vi "FW_PyRunAnnotaion.vi"(0 "Refnum in":refnum<k35>, 5 "python_image":u8[][][](array[numeric]), 9 "appended path":path, 11 "error in (no error)":errorcluster, 12 "Parameters in":T1={"scale_w"=0.0, "scale_h"=0.0, "offset_X"=0.0, "offset_Y"=0.0, "Rho"=0.0, "Theta"=0.0, "Threshold"=14, "min_line_len"=14, "max_line_gap"=30}) -> (1 "2D_image":u8[][](array[numeric]), 3 "elapsed time":u32, 4 "Refnum out":refnum<k35>, 6 "Python_img":u8[][][](array[numeric]), 8 "Lanes":cluster{"X":dbl, "Y":dbl}[][](array[cluster]), 10 "lines":cluster{"X":dbl, "Y":dbl}[][](array[cluster]), 14 "trapezoid_ROI":cluster{"X":dbl, "Y":dbl}[](array[cluster]), 15 "error out":errorcluster)   [LabVIEW 2021, in "Framework_lib.lvlib"]
uses:
  QMH/Framework_lib.lvlib
  FW_pyAnnotation_parameters.ctl
panel:
  out "return value":cluster{"out":dbl, "out 2":i32}
  out "Numeric":u32
  out "input size":cluster{"b":u32, "b":u32, "b":u32}
  # "[[[244 489 383 385]]\n\n [[223 489 380 384]]\n\n [[242 487 304 445]]\n\n [[292 454 370 396]]]"
  # "[[165, 539, 563, 259], []]"
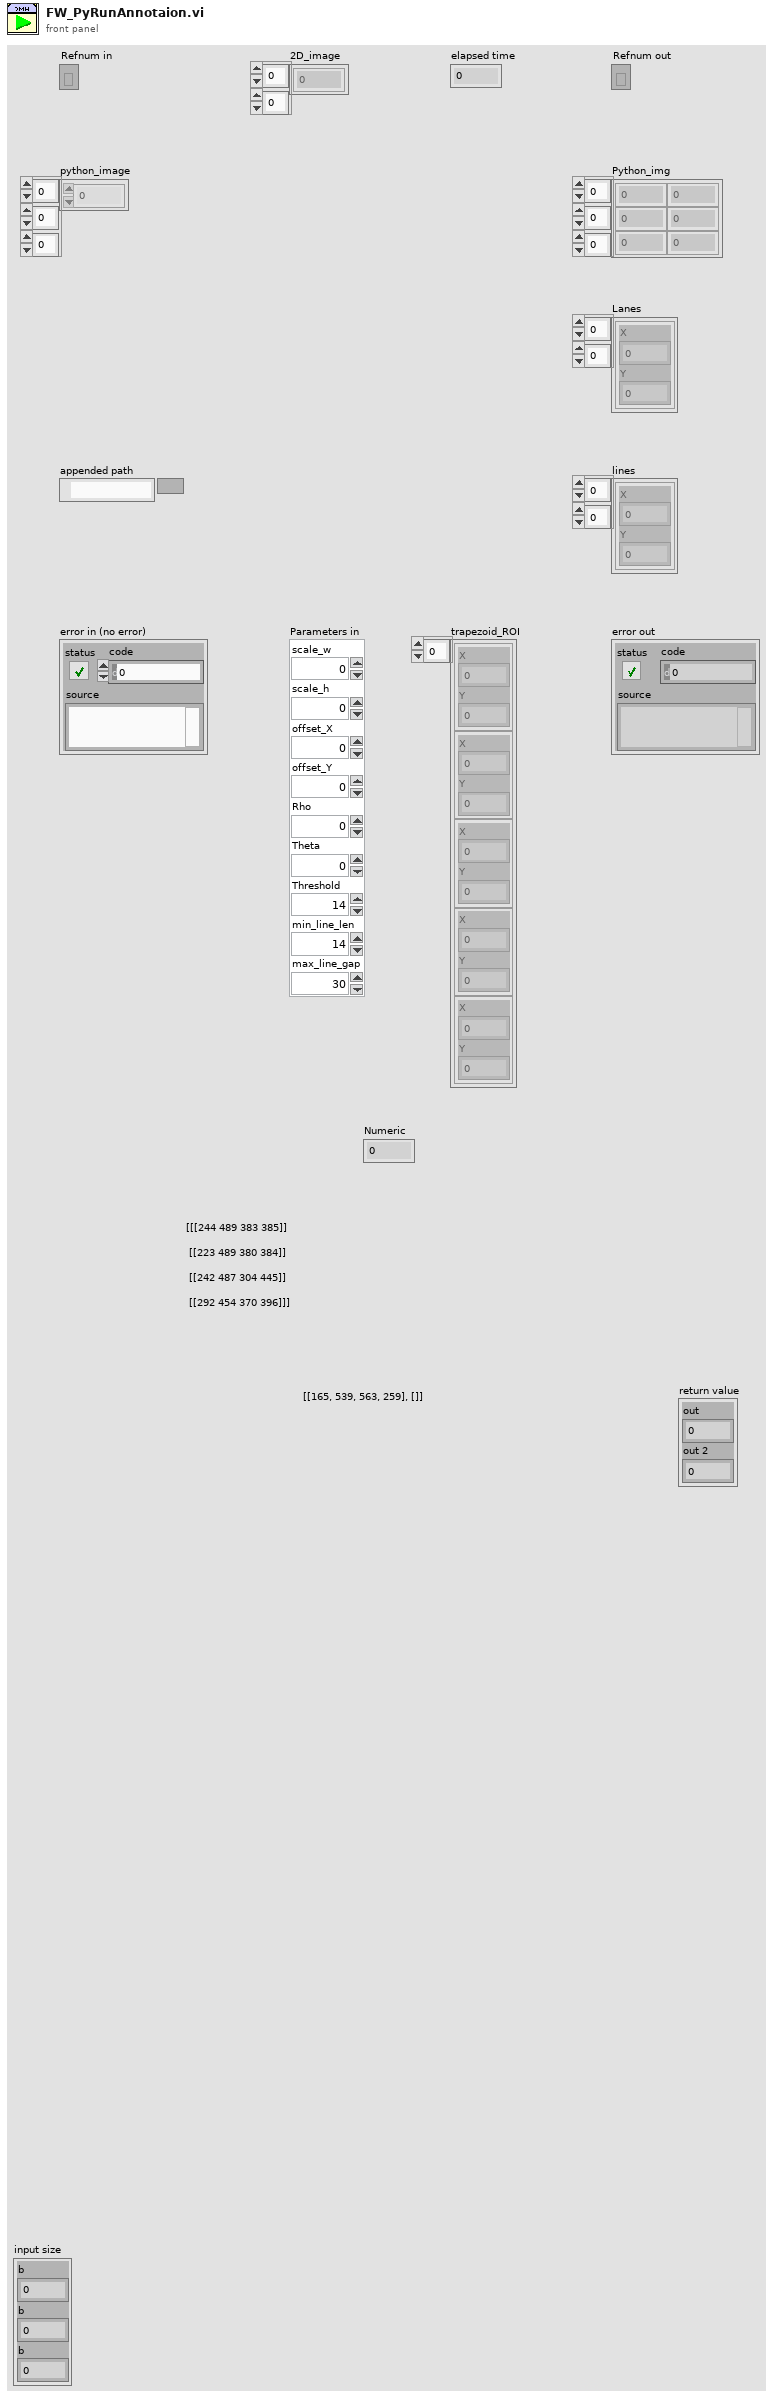
[diagram p1: front panel]
types:
  T1 = typedef "Framework_lib.lvlib/FW_pyAnnotation_parameters.ctl" = cluster{"scale_w":dbl, "scale_h":dbl, "offset_X":dbl, "offset_Y":dbl, "Rho":dbl, "Theta":dbl, "Threshold":i32, "min_line_len":i32, "max_line_gap":i32}
  T2 = cluster{"output":u8[][][], "vertices":i32[][][], "edges":u8[][], "Lines":i32[][][], "lanes":i32[][][]}
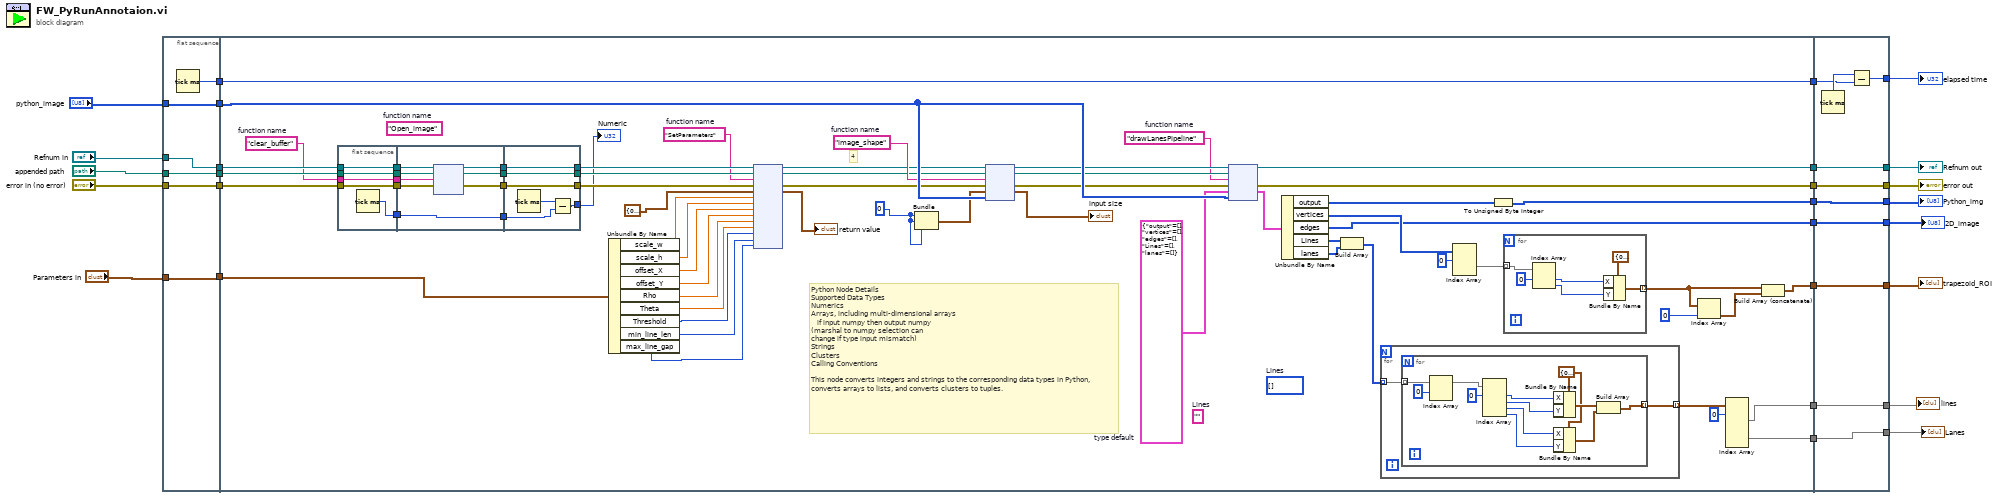
[diagram p0: block diagram]
diagram:
  n1 = flat-sequence {
    tunnel: "python_image" -> [w30]
    tunnel: "appended path" -> [w31]
    tunnel: "error in (no error)" -> [w32]
    tunnel: "Refnum in" -> [w33]
    tunnel: [w33] -> w27
    tunnel: [w32] -> w26
    tunnel: [w31] -> w25
    tunnel: [w30] -> w24
    tunnel: [w29] -> w23
    tunnel: [w28] -> w7
    tunnel: "Parameters in" -> [w28]
    tunnel: w27 -> [w97]
    tunnel: w26 -> [w96]
    tunnel: w25 -> [w93]
    tunnel: w24 -> [w92]
    tunnel: [w95] -> w22
    tunnel: [w94] -> w21
    tunnel: [w91] -> w20
    tunnel: w23 -> [w91]
    tunnel: [w90] -> w19
    tunnel: [w76] -> w18
    tunnel: [w35] -> w17
    tunnel: w7 -> [w59]
    tunnel: [w45] -> w4
    tunnel: [w34] -> w2
    tunnel: [w145] -> w15
    tunnel: [w146] -> w9
    tunnel: w22 -> [w146]
    tunnel: w21 -> [w145]
    tunnel: w20 -> [w143]
    tunnel: [w142] -> w11
    tunnel: [w141] -> w5
    tunnel: w19 -> [w141]
    tunnel: [w140] -> w13
    tunnel: w18 -> [w140]
    tunnel: [w139] -> w12
    tunnel: w17 -> [w139]
    tunnel: w4 -> [w138]
    tunnel: [w138] -> w3
    tunnel: w2 -> [w137]
    tunnel: [w137] -> w1
    frame #0 {
      n2 = Tick Count (ms)() -> (millisecond timer value=w29:u32)
    }
    frame #1 {
      (unwired) ""  # Lines
      (unwired) i32[] []  # Lines
      w58 = T2 {"output"=[], "vertices"=[], "edges"=[], "Lines"=[], "lanes"=[]}  # type default
      w66 = "SetParameters"  # function name
      w81 = "drawLanesPipeline"  # function name
      w85 = u32 0 ("b")
      w86 = "clear_buffer"  # function name
      (unwired) "Open_image"  # function name
      w89 = "image_shape"  # function name
      # "Python Node Details\nSupported Data Types\nNumerics\nArrays, including multi-dimensional arrays\n   if input numpy then output numpy\n(marshal to numpy selection can \nchange if type input mismatch)\nStrings\nClusters\nCalling Conventions\n\nThis node converts integers and strings to the corresponding data types in Python, converts arrays to lists, and converts clusters to tuples."
      # "4"
      n3 = flat-sequence {
        tunnel: w86 -> [w113]
        tunnel: w93 -> [w114]
        tunnel: w96 -> [w115]
        tunnel: w97 -> [w116]
        tunnel: [w116] -> w57
        tunnel: [w115] -> w56
        tunnel: [w114] -> w55
        tunnel: [w113] -> w54
        tunnel: [w112] -> w49
        tunnel: w57 -> [w124]
        tunnel: w56 -> [w123]
        tunnel: w55 -> [w122]
        tunnel: w54 -> [w120]
        tunnel: [w121] -> w53
        tunnel: [w119] -> w52
        tunnel: [w118] -> w51
        tunnel: [w117] -> w50
        tunnel: w49 -> [w117]
        tunnel: [w128] -> w68
        tunnel: [w129] -> w70
        tunnel: [w130] -> w87
        tunnel: w53 -> [w130]
        tunnel: w52 -> [w129]
        tunnel: w51 -> [w128]
        tunnel: w50 -> [w126]
        tunnel: [w125] -> w48
        frame #0 {
          n4 = Tick Count (ms)() -> (millisecond timer value=w112:u32)
        }
        frame #1 {
          n5 = node(w124, w122, w120, w123) -> (w119:refnum<k35>, w118:path, w121:errorcluster)  [unwired: 2 in, 1 out]
        }
        frame #2 {
          n6 = Tick Count (ms)() -> (millisecond timer value=w127:u32)
          n7 = Subtract(x=w127, y=w126) -> (x-y=w125:u32)
        }
      }
      n8 = Unbundle By Name(w59) -> ("scale_w"=w65:dbl, "scale_h"=w64:dbl, "offset_X"=w63:dbl, "offset_Y"=w62:dbl, "Rho"=w61:dbl, "Theta"=w44:dbl, "Threshold"=w43:i32, "min_line_len"=w42:i32, "max_line_gap"=w41:i32)
      n9 = node(w70, w68, w66, w87, cluster{"out":dbl, "out 2":i32} {"out"=0.0, "out 2"=0}, w65, w64, w63, w62, w61, w44, w43, w42, w41) -> (w69:refnum<k35>, w67:path, w71:errorcluster, →"return value":cluster{"out":dbl, "out 2":i32})  [unwired: 9 in, 1 out]
      n10 = Bundle("b"=w85, "b"=w85, "b"=w85) -> (w80:cluster{"b":u32, "b":u32, "b":u32})  [unwired: 1 in]
      n11 = node(w69, w67, w89, w71, w80, w92) -> (w83:refnum<k35>, w82:path, w88:errorcluster, →"input size":cluster{"b":u32, "b":u32, "b":u32})  [unwired: 1 in, 1 out]
      n12 = node(w83, w82, w81, w88, w58, w92) -> (w95:refnum<k35>, w94:errorcluster, w79:T2)  [unwired: 1 in, 2 out]
      n13 = Unbundle By Name(w79) -> ("output"=w46:u8[][][], "vertices"=w78:i32[][][], "edges"=w45:u8[][], "Lines"=w47:i32[][][], "lanes"=w37:i32[][][])
      n14 = Build Array(w47, w37) -> (w38:i32[][][][])
      n15 = for {
        tunnel: [w99] -> w72 mode=indexing
        tunnel: w38 -> [w98] mode=indexing
        n16 = for {
          tunnel: w98 -> [w108] mode=indexing
          tunnel: [w101] -> w99 mode=indexing
          w104 = cluster{"X":dbl, "Y":dbl} {"X"=0.0, "Y"=0.0} ("Point Coordinates")
          n17 = Index Array(array=w108, index (row)=0) -> (element=w107:i32[])  [unwired: 1 in]
          n18 = Index Array(array=w107, index #1=0 ("index")) -> (element #1=w110:i32, element #2=w111:i32, element #3=w103:i32, element #4=w102:i32)  [unwired: 3 in]
          n19 = Bundle By Name(cluster=w104, "X"=w110, "Y"=w111) -> (w105:cluster{"X":dbl, "Y":dbl})
          n20 = Bundle By Name(cluster=w104, "X"=w103, "Y"=w102) -> (w100:cluster{"X":dbl, "Y":dbl})
          n21 = Build Array(w105, w100) -> (w101:cluster{"X":dbl, "Y":dbl}[])
        }
      }
      n22 = Index Array(array=w78, index (dim 0)=0 ("index (page)")) -> (element=w60:i32[][])  [unwired: 2 in]
      n23 = To Unsigned Byte Integer(number=w46) -> (unsigned 8bit integer=w90:u8[][][])
      n24 = for {
        tunnel: w60 -> [w136] mode=indexing
        tunnel: [w131] -> w75 mode=indexing
        n25 = Index Array(array=w136, index #1=0 ("index")) -> (element #1=w133:i32, element #2=w132:i32)  [unwired: 1 in]
        n26 = Bundle By Name(cluster=cluster{"X":dbl, "Y":dbl} {"X"=0.0, "Y"=0.0} ("Point Coordinates"), "X"=w133, "Y"=w132) -> (w131:cluster{"X":dbl, "Y":dbl})
      }
      n27 = Index Array(array=w75, index=0) -> (element=w73:cluster{"X":dbl, "Y":dbl})
      n28 = Index Array(array=w72, index (dim 0) #1=0 ("index (page)")) -> (element #1=w35:cluster{"X":dbl, "Y":dbl}[][], element #2=w34:cluster{"X":dbl, "Y":dbl}[][])  [unwired: 5 in]
      n29 = Build Array (concatenate)(w75, w73) -> (w76:cluster{"X":dbl, "Y":dbl}[])
      "Numeric" <- w48
    }
    frame #2 {
      n30 = Tick Count (ms)() -> (millisecond timer value=w144:u32)
      n31 = Subtract(x=w144, y=w143) -> (x-y=w142:u32)
    }
  }
  "error out" <- w15
  "trapezoid_ROI" <- w13
  "lines" <- w12
  "Python_img" <- w5
  "elapsed time" <- w11
  "Refnum out" <- w9
  "2D_image" <- w3
  "Lanes" <- w1
